vi "Destroy.vi"(8 "error in":errorcluster, 11 "measurement service in":refnum<class "IMeasurement Service.lvclass">) -> (0 "error out":errorcluster)   [LabVIEW 2020, in "Plug-In SDK Measurement.lvlib" / "IMeasurement Service.lvclass"]
uses:
  IMeasurement Service.lvclass
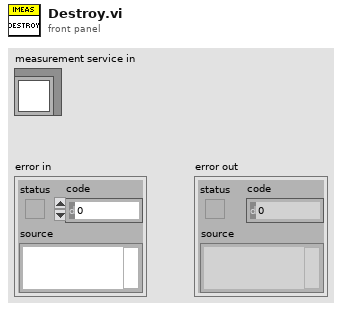
[diagram p1: front panel]
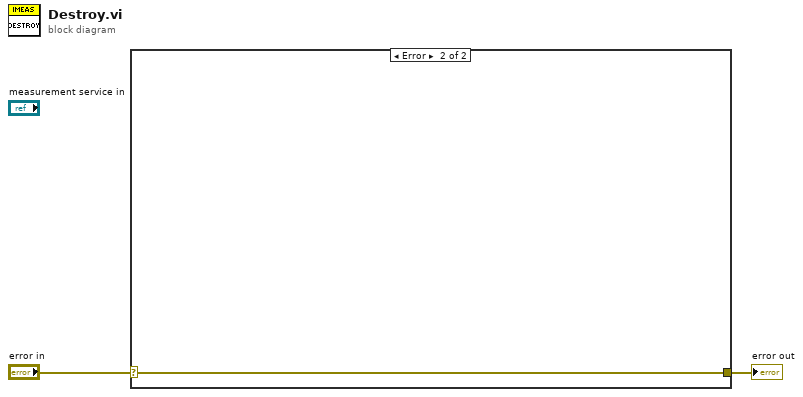
[diagram p0: block diagram]
diagram:
  n1 = case shown="Error" "error in" {
    selector: "error in" -> [w3 w4]
    tunnel: [w3 w4] -> w1
    frame No Error {
    }
    frame Error {
    }
  }
  "error out" <- w1
